vi "Write to Hardware.vi"(8 "error in (no error)":errorcluster, 10 "Values in":dbl[](array[numeric]), 11 "NI-XNET CAN Writer Execution Unit in":refnum<class "NI-XNET CAN Writer Execution Unit.lvclass">) -> (0 "error out":errorcluster, 2 "Values out":dbl[](array[numeric]), 3 "NI-XNET CAN Writer Execution Unit out":refnum<class "NI-XNET CAN Writer Execution Unit.lvclass">)   [LabVIEW 2020, in "Communication Bus Template Engine.lvlib" / "Implementation.lvlib" / "NI-XNET CAN Writer Execution Unit.lvclass"]
uses:
  NI-XNET CAN Writer Execution Unit.lvclass
  NI-XNET CAN Writer Execution Unit.lvclass/NI-XNET CAN Writer Execution Unit.ctl
  <vilib>/xnet/xnet.llb/XNET Write (Signal Single-point).vi
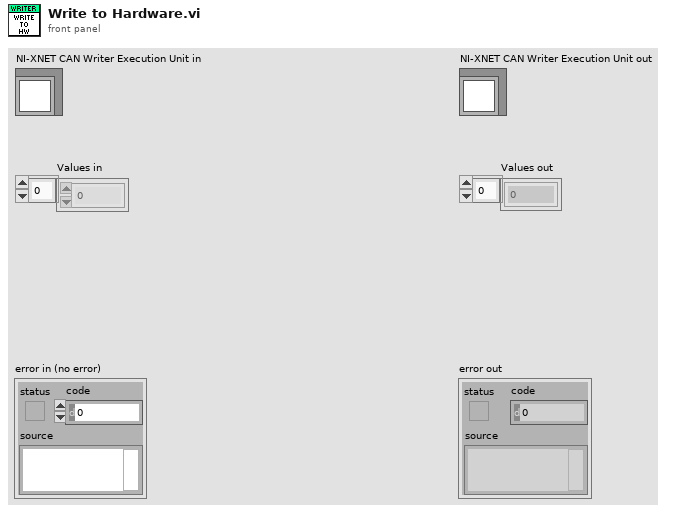
[diagram p1: front panel]
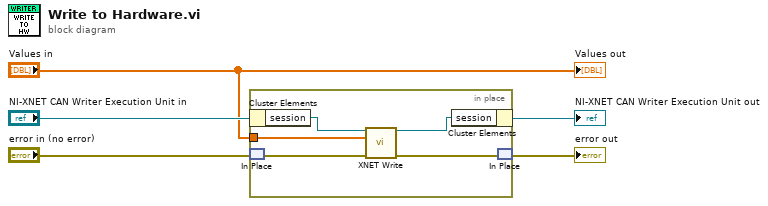
[diagram p0: block diagram]
diagram:
  n1 = in-place {
    in-place-border: "Values in" -> [w9]
    n2 = in-place-cluster #1("NI-XNET CAN Writer Execution Unit in") -> ("session"=w10:refnum<k21>)
    n3 = in-place-match #2("error in (no error)") -> (w7:errorcluster)
    n4 = call-poly <vilib>:"XNET Write.vi"("session in"=w10, "data"=w9, "error in (no error)"=w7) -> ("session out"=w6:refnum<k21>, "error out"=w8:errorcluster)  [unwired: 11 in]
    n5 = in-place-cluster #1("session"=w6) -> (→"NI-XNET CAN Writer Execution Unit out":refnum<class "NI-XNET CAN Writer Execution Unit.lvclass">)
    n6 = in-place-match #2(w8) -> (→"error out":errorcluster)
  }
  "Values out" <- "Values in"
